vi "Dashboard.Main.vi"() -> ()   [LabVIEW 2014]
uses:
  <vilib>/event_ctls.llb/eventvkey.ctl
  <vilib>/Rock Robotics/WPI/Dashboard/WPI_DashboardLogging Global.vi
  <vilib>/Rock Robotics/Network Tables/SD Read Number.vi
  <vilib>/Rock Robotics/Network Tables/SD Read String.vi
  <vilib>/Rock Robotics/Network Tables/SD Read Boolean.vi
  <vilib>/Rock Robotics/Network Tables/SD Write Number.vi
  <vilib>/Utility/config.llb/Write Key (String).vi
  <vilib>/Utility/config.llb/Write Key (I32).vi
  <vilib>/Utility/config.llb/NI_LVConfig.lvlib
panel:
  in  "TCP":refnum<k5>
  in  "Rec Mode":enum32{"Stop", "Record", "Playback"}(radio)
  in  "Vision":u16(ring) items=["Camera Off", "USB Camera SW", "USB Camera HW", "IP Camera"]
  out "Camera IP":string
  out "Image Message":string="Timeout in Camera Communications"
  in  "Dashboard Tab":T1(tab)=enum."Auto"
  in  "Camera Settings":T2={"Frame Rate"=30, "Compression"=30, "Size"=1} {"Frame Rate" scale=1.0..30.0; "Size" items=["640x480", "320x240", "160x120"]}
  out "MotorChart R":cluster{"Numeric":dbl, "Numeric":dbl}(graph)
  out "MotorChart L":T3(graph)
  out "MotorSliders R":cluster{"MotorSlide1":dbl, "MotorSlide2":dbl} {"MotorSlide2" scale=-1.0..1.0 scale format="%#_2e"; "MotorSlide1" scale=-1.0..1.0 scale format="%#_2e"}
  out "MotorSliders L":T4 {"MotorSlide4 2" scale=0.0..14.0 scale format="%#_2e"; "MotorSlide2" scale=-1.0..1.0 scale format="%#_2e"; "MotorSlide1" scale=-1.0..1.0 scale format="%#_2e"}
  out "Gyro":dbl(knob) scale=0.0..360.0
  out "JS1 Z":dbl(slide) scale=-1.0..1.0 scale format="%#_2e"
  out "JS1 Graph":cluster{"X":dbl, "Y":dbl}[](graph)
  out "JS1 Buttons":T5
  out "JS2 Z":dbl(slide) scale=-1.0..1.0 scale format="%#_2e"
  out "JS2 Graph":cluster{"X":dbl, "Y":dbl}[](graph)
  out "JS2 Buttons":T5
  out "Mode":T6(ring)=enum."Auto Disabled"
  in  "DB Camera Config":bool
  out "fps":dbl format="%#.1g"
  out "Mbps":dbl format="%#.1g"
  out "Mbps 2":bool
  out "Front Detector":bool
  out "Stacker Position":dbl(slide) scale=0.0..20.0
  out "Rear Detector":bool
  out "Current Angle":dbl(knob) scale=0.0..360.0
  out "Commanded Heading":dbl(knob) scale=0.0..360.0
  in  "Auto Selection":T7(radio)
  out "Callback":string
  in  "DB/String 9":string
  in  "DB/String 8":string
  in  "DB/String 7":string
  in  "DB/String 6":string
  in  "DB/String 5":string
  in  "DB/String 4":string
  in  "DB/String 3":string
  in  "DB/String 2":string
  in  "DB/String 1":string
  in  "DB/String 0":string
  in  "DB/Slider 0":dbl(slide) scale=0.0..5.0
  in  "DB/Slider 1":dbl(slide) scale=0.0..5.0
  in  "DB/Slider 2":dbl(slide) scale=0.0..5.0
  in  "DB/Slider 3":dbl(slide) scale=0.0..5.0
  out "DB/LED 3":bool
  out "DB/LED 2":bool
  out "DB/LED 1":bool
  out "DB/LED 0":bool
  in  "DB/Button 3":bool
  in  "DB/Button 2":bool
  in  "DB/Button 1":bool
  in  "DB/Button 0":bool caption="New Name"
  in  "Test Slider":dbl(slide) scale=0.0..100.0 scale format="%#_3g"
  in  "On/Off":bool caption="Solenoid"
  in  "Test Name":u16(ring) items=["Select the test to run...", "Example Test", "-------------------------------", "List of tests is built in robot code.", "Replace with your own automated tests."]
  in  "Test Tree":string(tree)
  in  "Motor":cluster{"Value":dbl, "Enable":bool} {"Value" scale=-1.0..1.0 scale format="%#_3g"}
  out "Progress":T8 {"Test Progress" scale=0.0..100.0}
  in  "Rev/Fwd":cluster{"Forward":bool, "Reverse":bool}
  in  "Test Ring":u16(ring) items=["Monochrome", "Color"]
  in  "Listbox":i32(listbox)
  out "Tree":string(tree)
  out "Camera Image":T9(plugin-control)
  out "Boolean":bool
  # "Left"
  # "Front"
  # "Right"
  # "Battery"
  # "Primary"
  # "Secondary"
  # "Development"
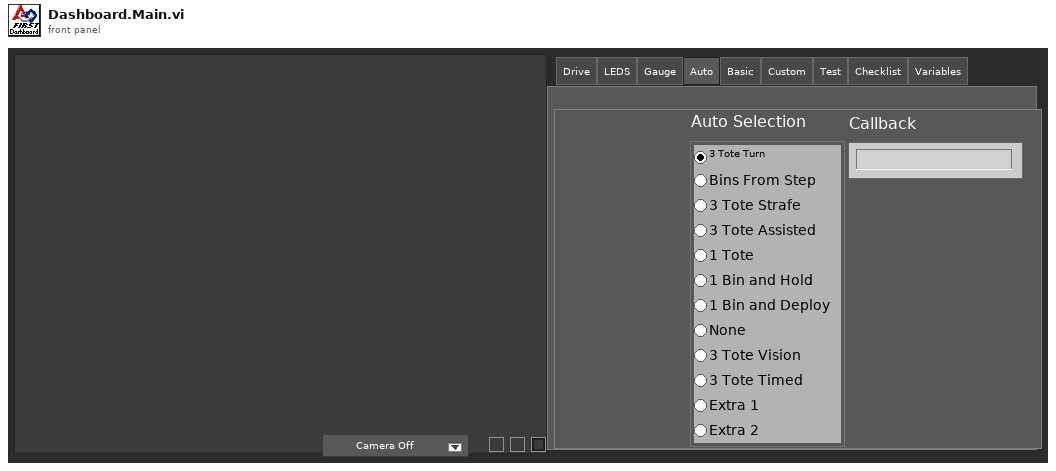
[diagram p1: front panel]
types:
  T1 = enum32{"Drive", "LEDS", "Gauge", "Auto", "Basic", "Custom", "Test", "Checklist", "Variables"}
  T2 = cluster{"Frame Rate":i32, "Compression":i32, "Size":u16}
  T3 = cluster{"Numeric":dbl, "Numeric":dbl, "Battery V":dbl}
  T4 = cluster{"MotorSlide1":dbl, "MotorSlide2":dbl, "MotorSlide4 2":dbl}
  T5 = cluster{bool, bool, bool, bool, bool, bool, bool, bool, bool, bool, bool, bool}
  T6 = enum8{"Tele-Op Disabled", "Tele-Op Enabled", "Auto Disabled", "Auto Enabled", "Test Disabled", "Test Enabled", "Disconnected", "No Code", "E-Stop"}
  T7 = enum32{"3 Tote Turn", "Bins From Step", "3 Tote Strafe", "3 Tote Assisted", "1 Tote", "1 Bin and Hold", "1 Bin and Deploy", "None", "3 Tote Vision", "3 Tote Timed", "Extra 1", "Extra 2"}
  T8 = cluster{"Test Progress":u8, "Test Progress Text":string}
  T9 = typedef "IMAQ Image.ctl" = refnum<image>
  T10 = enum32{"Drive", "Basic", "Custom", "Test", "Checklist", "Variables"}
  T11 = typedef "Image Type" = u32
  T12 = cluster{"Camera Image":refnum<vi>, "Dashboard Tab":refnum<vi>, "Boolean":refnum<vi>, "Vision":refnum<vi>, "Rec Mode":refnum<vi>, "Test Slider":refnum<vi>, "On/Off ":refnum<vi>, "Test Ring":refnum<vi>, "Rev/Fwd":refnum<vi>, "Test Name":refnum<vi>, "Motor":refnum<vi>, "Progress":refnum<vi>, "CheckList":refnum<vi>, "Tree":refnum<vi>, "Test Tree":refnum<vi>}
  T13 = typedef "NI_LVConfig.lvlib/Config Data RefNum.ctl" = refnum<k1>
  T14 = cluster{"Error Strings":string, "Disable Counts":cluster{u16, u16}, "Rail Faults":cluster{u16, u16, u16}, "Robot IP":string, "DB Mode":u8, "Event Info":cluster{"Name":string, "Type":u8, "Number":u16, "Replay":u8}, "Camera Addr":string}
  T15 = cluster{"Storage":cluster{"Disk Free":u64, "RAM Block":u32, "RAM free":u32}, "CPU Utilization":cluster{"CPU % ISR":sgl, "CPU % Time Crit":sgl, "CPU % Timed Str":sgl, "CPU % High":sgl, "CPU % Above":sgl, "CPU % Normal":sgl, "CPU % Low":sgl}, "CAN":cluster{"% Bus Utilization":sgl, "Bus Off Cnt":u32, "TX_FIFO Full Cnt":u32, "Receive Error Cnt":u8, "Transmit Error Cnt":u8}, "HID":cluster{"HID Outputs":u32, "Rumble Low":u16, "Rumble High":u16}[]}
  T16 = cluster{"Status bits":cluster{"Test Mode":bool, "Autonomous":bool, "Enabled":bool, "Code Start":bool, "Brownout":bool, "Reserved 2":bool, "Reserved 3":bool, "E-Stop":bool}, "Code Trace":cluster{"Disabled":bool, "TeleOp":bool, "Auto":bool, "Test":bool}, "Controller Type":enum16{"unknown", "cRIO", "roboRio"}, "Code?":enum16{"unknown", "noCode", "code"}, "Battery V":dbl}
  T17 = cluster{"Control Bits":cluster{"TestMode":bool, "Autonomous":bool, "Enabled":bool, "FMS Present":bool, bool, bool, bool, "E-Stop":bool}, "Team Station ":u8, "Countdown":sgl, "Joystick Values":cluster{"Axes":dbl[], "Buttons":bool[], "POVs":i16[]}[]}
  T18 = cluster{"Axes":dbl[], "Buttons":bool[], "POVs":i16[]}[]
  T19 = cluster{"Axes":dbl[], "Buttons":bool[], "POVs":i16[]}
  T20 = cluster{"Buttons[0]":bool, "Buttons[1]":bool, "Buttons[2]":bool, "Buttons[3]":bool, "Buttons[4]":bool, "Buttons[5]":bool, "Buttons[6]":bool, "Buttons[7]":bool, "Buttons[8]":bool, "Buttons[9]":bool, "Buttons[10]":bool, "Buttons[11]":bool}
  T21 = cluster{"Operation":enum16{"Update", "Clear"}, "Color Box":u32}[]
  T22 = typedef "eventvkey.ctl" = enum16{"ASCII", "Enter", "Return", "Shift", "Ctrl", "Alt", "Cmd", "Opt", "Caps", "NumLock", "Clear", "Break", "Up", "Down", "Left", "Right", "Insert", "Delete", "Home", "End", "PageUp", "PageDown", "Escape", "Help", "Pause", "ScrollLock", "F1", "F2", "F3", "F4", "F5", "F6", "F7", "F8", "F9", "F10", "F11", "F12", "F13", "F14", "F15", "F16", "F17", "F18", "F19", "F20", "F21", "F22", "F23", "F24", "Play", "VolumeUp", "VolumeDown", "Mute", "Two Byte Char"}
  T23 = cluster{"Image Size":bool, "Image Type":bool, "Pixel Value":bool, "ROI Information":bool, "Zoom Factor":bool}
  T24 = enum8{"Enabled", "Disabled", "Disabled and Grayed Out"}
  T25 = cluster{"Operation":enum16{"Update", "Clear"}, "Color Box":u32}
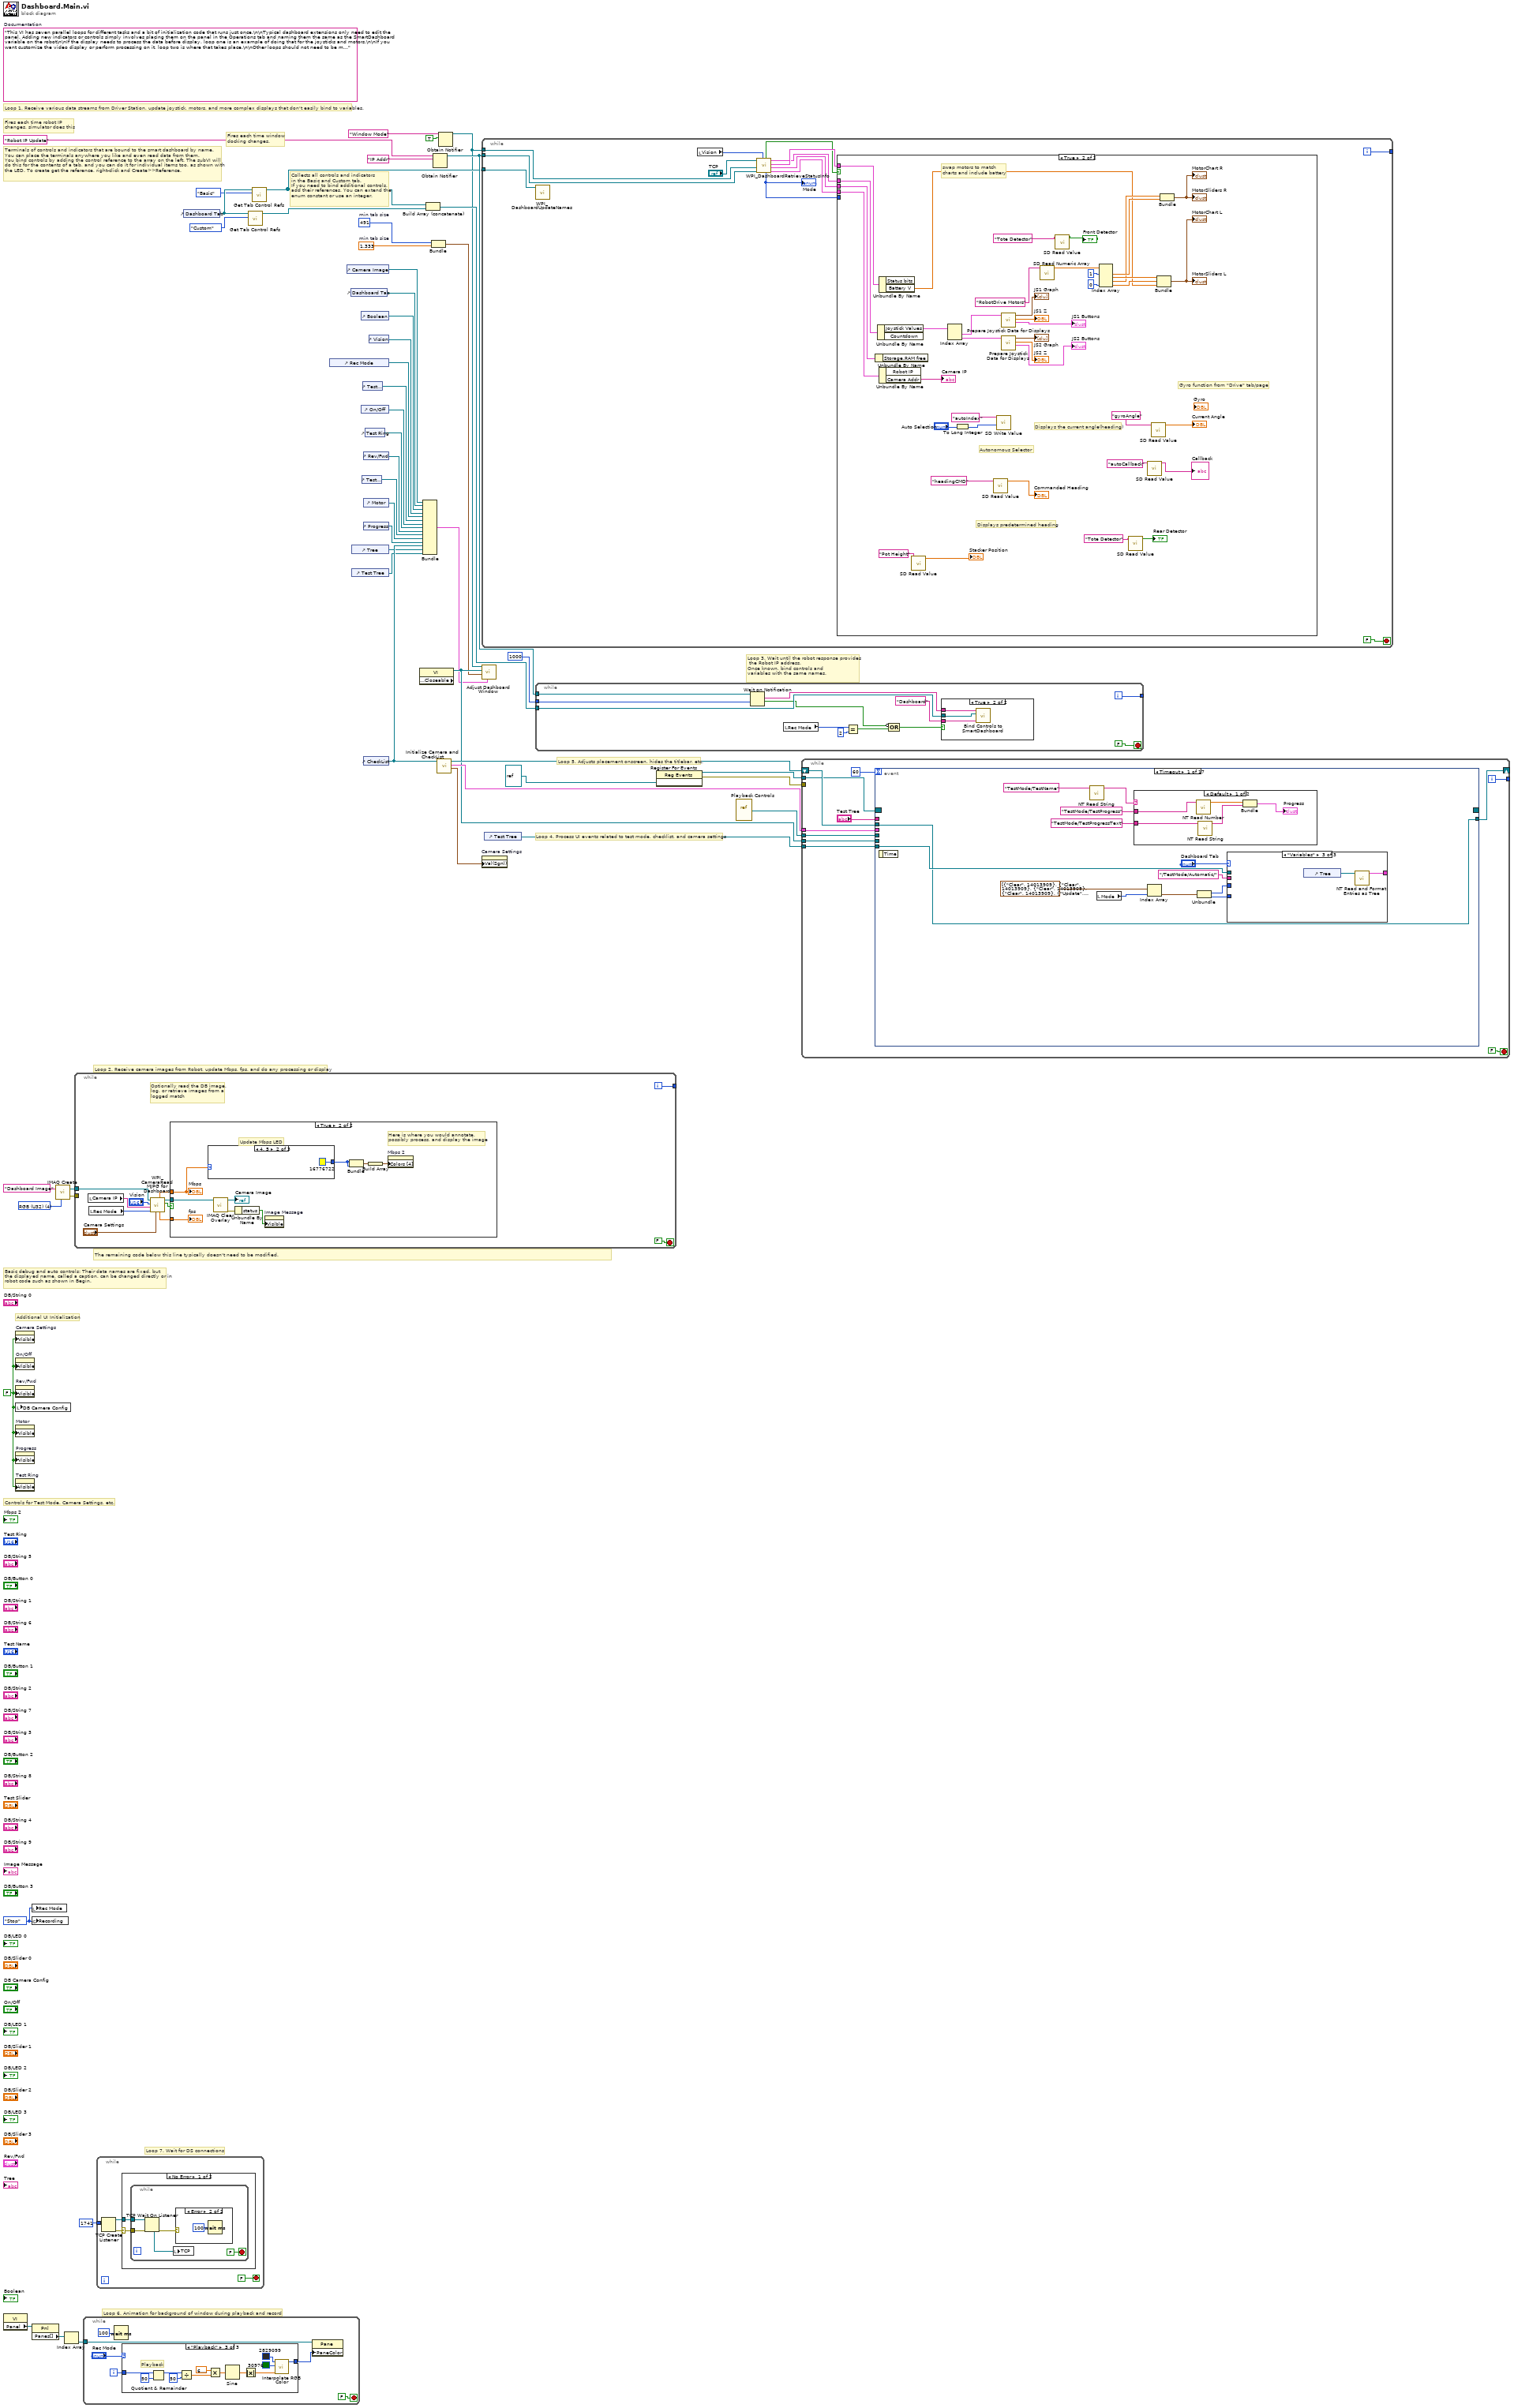
[diagram p0: block diagram]
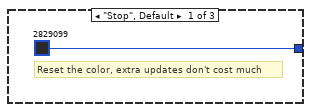
[diagram p5: hidden frame]
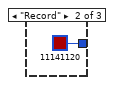
[diagram p6: hidden frame]
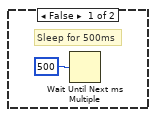
[diagram p8: hidden frame]
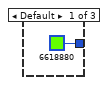
[diagram p9: hidden frame]
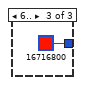
[diagram p10: hidden frame]
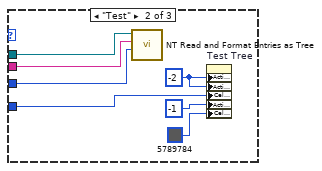
[diagram p12: hidden frame]
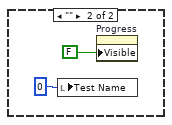
[diagram p13: hidden frame]
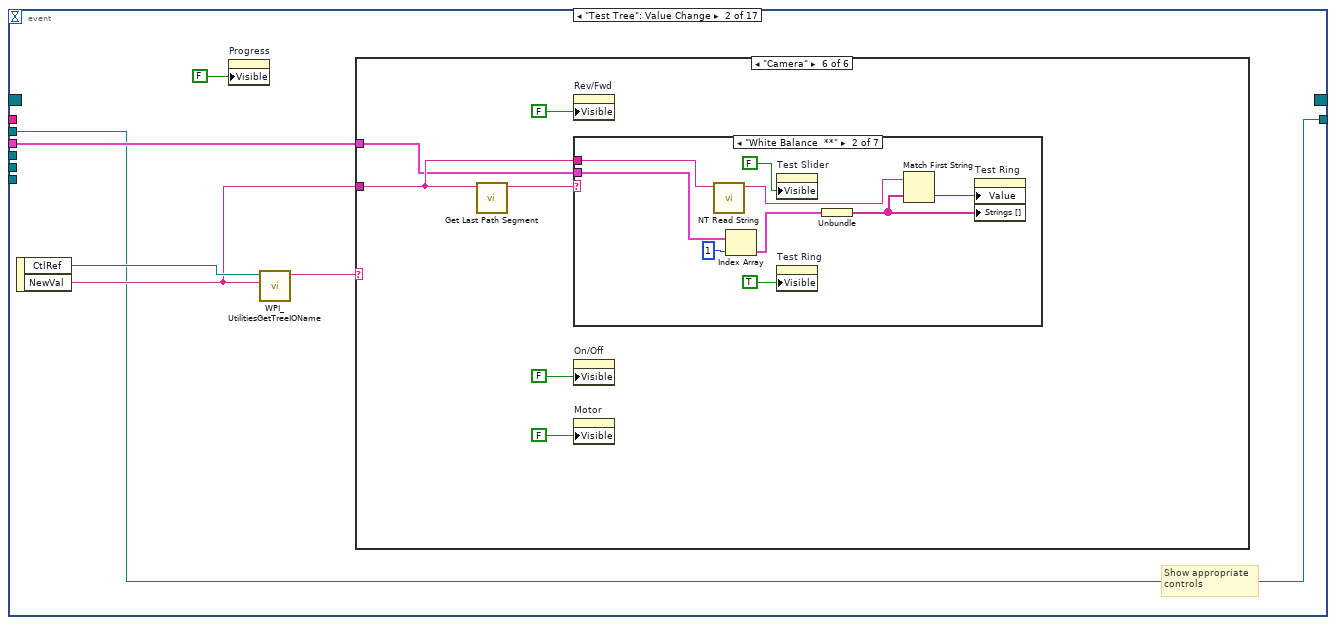
[diagram p14: hidden frame]
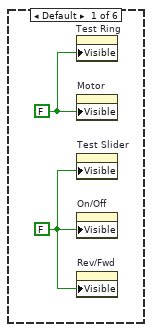
[diagram p15: hidden frame]
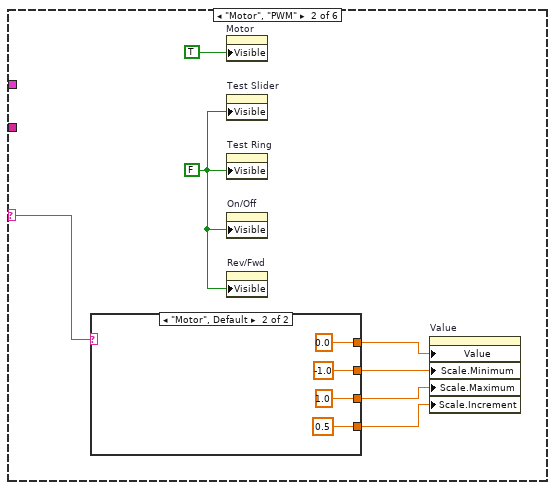
[diagram p16: hidden frame]
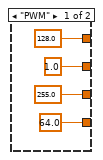
[diagram p17: hidden frame]
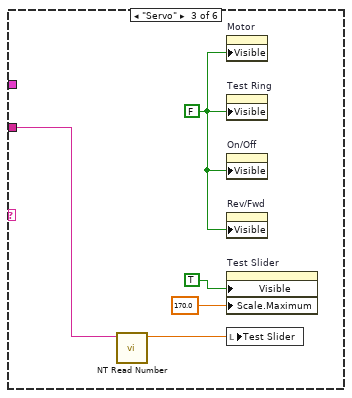
[diagram p18: hidden frame]
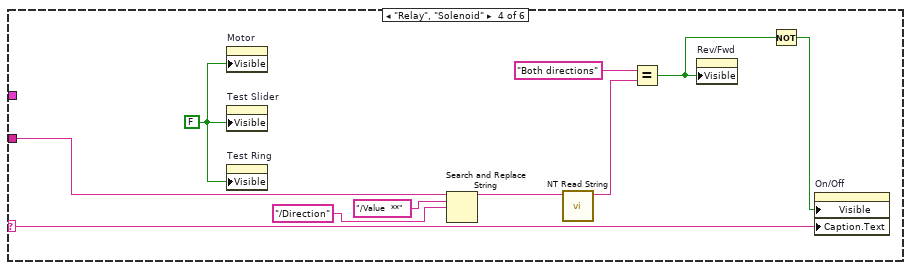
[diagram p19: hidden frame]
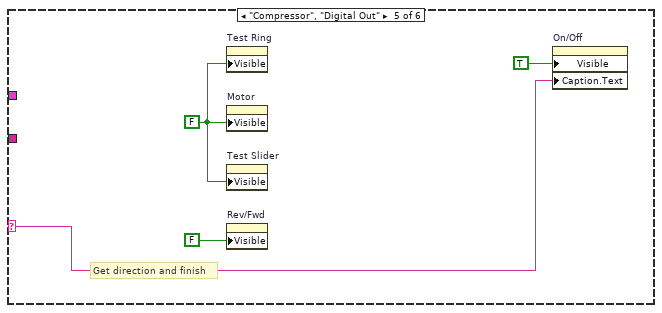
[diagram p20: hidden frame]
diagram:
  w23 = 491  # min tab size
  w22 = 1.333  # min tab size
  w31 = enum32{"Stop", "Record", "Playback"}."Stop" ("Rec Mode")
  w5 = FALSE ("Visible")
  (unwired) "This VI has seven parallel loops for different tasks and a bit of initialization code that runs just once.\n\nTypical dashboard extensions only need to edit the panel. Adding new indicators or controls simply involves placing them on the panel in the Operations tab and naming them the same as the SmartDashboard variable on the robot\n\nIf the display needs to process the data before display, loop one is an example of doing that for the joysticks and motors.\n\nIf you want customize the video display or perform processing on it, loop two is where that takes place.\n\nOther loops should not need to be modified. They are pretty standard, and document the task they perform."  # Documentation
  w51 = T11 4 items=["Grayscale (U8)", "Grayscale (I16)", "Grayscale (SGL)", "Complex (CSG)", "RGB (U32)", "HSL (U32)", "RGB (U64)"] ("Image Type")
  # "Loop 7. Wait for DS connections"
  # "Basic debug and auto controls: Their data names are fixed, but\nthe displayed name, called a caption, can be changed directly or in\nrobot code such as shown in Begin."
  # "Controls for Test Mode, Camera Settings, etc."
  # "Additional UI Initialization"
  # "Loop 6. Animation for background of window during playback and record"
  # "Fires each time robot IP\nchanges, simulator does this"
  # "Fires each time window\ndocking changes."
  # "Collects all controls and indicators\nin the Basic and Custom tab.\nIf you need to bind additional controls,\nadd their references. You can extend the\nenum constant or use an integer."
  # "The remaining code below this line typically doesn't need to be modified."
  # "Loop 4. Process UI events related to test mode, checklist, and camera settings"
  # "Terminals of controls and indicators that are bound to the smart dashboard by name.\nYou can place the terminals anywhere you like and even read data from them.\nYou bind controls by adding the control reference to the array on the left. The subVI will\ndo this for the contents of a tab, and you can do it for individual items too, as shown with\nthe LED. To create get the reference, right-click and Create>>Reference."
  # "Loop 3. Wait until the robot response provides\n the Robot IP address.\nOnce known, bind controls and\nvariables with the same names."
  # "Loop 5. Adjusts placement onscreen, hides the titlebar, etc."
  # "Loop 1. Receive various data streams from Driver Station, update joystick, motors, and more complex displays that don't easily bind to variables."
  # "Loop 2. Receive camera images from Robot, update Mbps, fps, and do any processing or display"
  n1 = property class="VI"() -> ("Panel"=w38:refnum<vi>)  [unwired: 2 in, 2 out]
  n2 = property on="Camera Settings" class="Clust (strict)"("Visible"=w5) -> ()  [unwired: 2 in, 2 out]
  n3 = property on="On/Off" class="Bool (strict)"("Visible"=w5) -> ()  [unwired: 2 in, 2 out]
  n4 = property on="Rev/Fwd" class="Clust (strict)"("Visible"=w5) -> ()  [unwired: 2 in, 2 out]
  n5 = local write "DB Camera Config"(w5) -> ()
  n6 = property on="Motor" class="Clust (strict)"("Visible"=w5) -> ()  [unwired: 2 in, 2 out]
  n7 = property on="Progress" class="Clust (strict)"("Visible"=w5) -> ()  [unwired: 2 in, 2 out]
  n8 = property on="Test Ring" class="Ring (strict)"("Visible"=w5) -> ()  [unwired: 2 in, 2 out]
  n9 = local write "Rec Mode"(w31) -> ()
  n10 = global write "WPI_DashboardLogging Global.vi" "Recording"(w31) -> ()
  n11 = property class="Pnl"(reference=w38) -> ("Panes[]"=w39:refnum<vi>[])  [unwired: 1 in, 2 out]
  n12 = call "IMAQ Create"("Image Name"="Dashboard Image", "Image Type"=w51) -> ("New Image"=w49:T9, "error out"=w48:errorcluster)  [unwired: 2 in, 1 out]
  n13 = Index Array(array=w39) -> (element=w37:refnum<vi>)  [unwired: 1 in]
  n14 = while {
    tunnel: w49 -> [w60]
    tunnel: w48 -> [_]
    tunnel: [w61] -> _
    i -> [w61]
    stop <- FALSE stop-if-true
    # "Optionally read the DB image,\nlog, or retrieve images from a\nlogged match"
    n15 = local read "Camera IP"() -> (w52:string)
    n16 = local read "Rec Mode"() -> (w54:enum32{"Stop", "Record", "Playback"})
    n17 = call <vilib>:"WPI_CameraRead MJPG for Dashboard.vi"("Camera Settings"="Camera Settings", "Rec Mode"=w54, "Camera IP"=w52, "Camera Mode"="Vision", "Refnum in"=w60) -> ("Active"=w58:bool, "Refnum out"=w59:T9, "FPS"=w57:dbl, "Bandwidth (Mbps)"=w56:dbl)  [unwired: 3 in]
    n18 = case shown="True" w58 {
      tunnel: w59 -> [_ w67]
      tunnel: w56 -> [_ w66]
      tunnel: w57 -> [_ w64]
      frame False {
        # "Sleep for 500ms"
        n19 = Wait Until Next ms Multiple(millisecond multiple=u32 500) -> ()  [unwired: 1 out]
      }
      frame True {
        # "Here is where you would annotate,\npossibly process, and display the image"
        # "Update Mbps LED"
        n20 = case shown="4, 5" w66 {
          tunnel: [u32 6618880 ("Color Box") u32 16776722 ("Color Box") u32 16716800 ("Color Box")] -> w68
          frame Default {
          }
          frame 4, 5 {
          }
          frame 6.. {
          }
        }
        n21 = call "IMAQ Clear Overlay"("Image"=w67) -> ("error out"=w71:errorcluster, "Image Out"=→"Camera Image":T9)  [unwired: 2 in, 7 out]
        n22 = Unbundle By Name(w71) -> ("status"=w72:bool)
        n23 = property on="Image Message" class="Str"("Visible"=w72) -> ()  [unwired: 2 in, 2 out]
        n24 = Bundle("Color Box"=w68, "Color Box"=w68) -> (w70:cluster{"Color Box":u32, "Color Box":u32})  [unwired: 1 out]
        n25 = Build Array(w70) -> (w69:cluster{"Color Box":u32, "Color Box":u32}[])
        n26 = property on="Mbps 2" class="Bool (strict)"("Colors [4]"=w69) -> ()  [unwired: 2 in, 2 out]
        "Mbps" <- w66
        "fps" <- w64
      }
    }
  }
  n27 = while {
    tunnel: w37 -> [w77]
    i -> [w80]
    stop <- FALSE stop-if-true
    n28 = Wait (ms)(milliseconds to wait=u32 100) -> ()  [unwired: 1 out]
    n29 = case shown="\"Playback\"" "Rec Mode" {
      tunnel: w80 -> [_ _ w95]
      tunnel: [u32 2829099 ("Base Color") u32 11141120 ("Target Color") w84] -> w76
      frame "Stop", Default {
        # "Reset the color, extra updates don't cost much"
      }
      frame "Record" {
      }
      frame "Playback" {
        # "Playback"
        n30 = Quotient & Remainder(x=w95, y=u32 50 ("milliseconds to wait")) -> (x-y*floor(x/y)=w91:u32)  [unwired: 1 out]
        n31 = Divide(x=w91, y=u32 50 ("milliseconds to wait")) -> (x/y=w88:dbl)
        n32 = Multiply(x=6.283185307179586, y=w88) -> (x*y=w93:dbl)
        n33 = Sine(x=w93) -> (sin(x)=w92:dbl)
        n34 = Absolute Value(x=w92) -> (abs(x)=w85:dbl)
        n35 = call "Interpolate RGB Color.vi"("Proportion"=w85, "Target Color"=u32 30976, "Base Color"=u32 2829099) -> ("Result Color"=w84:u32)  [unwired: 8 in]
      }
    }
    n36 = property class="Pane"(reference=w77, "PaneColor"=w76) -> ()  [unwired: 1 in, 2 out]
  }
  n37 = while {
    tunnel: u16 1741 ("timeout ms (25000)") -> [w99]
    stop <- FALSE stop-if-true
    n38 = TCP Create Listener(10:w99) -> (0:w96:errorcluster, 3:w98:refnum<k5>)  [unwired: 4 in, 1 out]
    n39 = case shown="No Error" w96 {
      selector: w96 -> [w100 _]
      tunnel: w98 -> [w101 _]
      frame No Error {
        n40 = while {
          tunnel: w101 -> [w105]
          tunnel: w100 -> [w103]
          stop <- FALSE stop-if-true
          n41 = TCP Wait On Listener(8:w103, 11:w105) -> (0:w102:errorcluster, 4:w104:refnum<k5>)  [unwired: 2 in, 3 out]
          n42 = local write "TCP"(w104) -> ()
          n43 = case shown="Error" w102 {
            frame No Error {
            }
            frame Error {
              n44 = Wait (ms)(milliseconds to wait=u32 100) -> ()  [unwired: 1 out]
            }
          }
        }
      }
      frame Error {
      }
    }
  }
  n45 = control-ref of="Dashboard Tab"() -> (w29:refnum<vi>)
  n46 = call <vilib>:"Get Tab Control Refs.vi"("Page Index"=T10."Custom" ("Dashboard Tab"), "TabControl in"=w29) -> ("ControlsOnPage"=w28:refnum<vi>[])  [unwired: 9 in]
  n47 = call <vilib>:"Get Tab Control Refs.vi"("Page Index"=T10."Basic" ("Dashboard Tab"), "TabControl in"=w29) -> ("ControlsOnPage"=w3:refnum<vi>[])  [unwired: 9 in]
  n48 = control-ref of="Rec Mode"() -> (w11:refnum<vi>)
  n49 = control-ref of="Camera Image"() -> (w26:refnum<vi>)
  n50 = control-ref of="Dashboard Tab"() -> (w25:refnum<vi>)
  n51 = control-ref of="Tree"() -> (w15:refnum<vi>)
  n52 = control-ref of="Test Tree"() -> (w14:refnum<vi>)
  n53 = control-ref of="Boolean"() -> (w20:refnum<vi>)
  n54 = control-ref of="On/Off"() -> (w9:refnum<vi>)
  n55 = control-ref of="Test Name"() -> (w13:refnum<vi>)
  n56 = control-ref of="Test Slider"() -> (w10:refnum<vi>)
  n57 = control-ref of="Rev/Fwd"() -> (w7:refnum<vi>)
  n58 = control-ref of="Motor"() -> (w12:refnum<vi>)
  n59 = control-ref of="Progress"() -> (w6:refnum<vi>)
  n60 = control-ref of="CheckList"() -> (w16:refnum<vi>)
  n61 = control-ref of="Test Ring"() -> (w8:refnum<vi>)
  n62 = control-ref of="Vision"() -> (w24:refnum<vi>)
  n63 = property class="VI" props=["Front Panel.Closeable"]() -> (reference out=w30:refnum<vi>)  [unwired: 2 in, 2 out]
  n64 = Bundle("Camera Image"=w26, "Dashboard Tab"=w25, "Boolean"=w20, "Vision"=w24, "Rec Mode"=w11, "Test Slider"=w10, "On/Off"=w9, "Test Ring"=w8, "Rev/Fwd"=w7, "Test Name"=w13, "Motor"=w12, "Progress"=w6, "CheckList"=w16, "Tree"=w15, "Test Tree"=w14) -> (w17:T12)  [unwired: 1 in]
  n65 = Build Array (concatenate)(w3, w28) -> (w27:refnum<vi>[])
  n66 = Bundle("min tab size"=w23, "min tab size"=w22) -> (w21:cluster{"min tab size":i32, "min tab size":dbl})  [unwired: 1 in]
  n67 = Obtain Notifier(name (unnamed)="Robot IP Update", notification data type="IP Addr" ("name (unnamed)")) -> (notifier out=w4:refnum<notifier>)  [unwired: 2 in, 2 out]
  n68 = call "Initialize Camera and CheckList.vi"("ListBox in"=w16) -> ("Cluster"=w42:cluster{"value":i32, "value":i32, "index":i32}, "Array"=w43:cluster{string[]}[], "File Refnum"=w41:T13)  [unwired: 8 in]
  n69 = Obtain Notifier(name (unnamed)="Window Mode", notification data type=TRUE) -> (notifier out=w2:refnum<notifier>)  [unwired: 2 in, 2 out]
  n70 = while {
    tunnel: [w119] -> _
    tunnel: w4 -> [w113]
    tunnel: w3 -> [w112]
    tunnel: w2 -> [w108]
    i -> [w119]
    stop <- FALSE stop-if-true
    n71 = call <vilib>:"WPI_DashboardUpdateNames.vi"("Controls on Tab"=w112) -> ()  [unwired: 11 in]
    n72 = local read "Vision"() -> (w110:u16)
    n73 = call <vilib>:"WPI_DashboardRetrieveStatusInfo.vi"("Vision"=w110, "Binding Refnum"=w113, "Window Mode Notifier"=w108, "TCP Cnx"="TCP") -> ("Power and Errors"=w114:T14, "Robot Metrics"=w117:T15, "Status Info"=w118:T16, "Control Info"=w115:T17, "Robot Mode"=w111:T6, "Process?"=w116:bool)  [unwired: 2 in]
    "Mode" <- w111
    n74 = case shown="True" w116 {
      tunnel: w118 -> [_ w160]
      tunnel: w117 -> [_ w159]
      tunnel: w115 -> [_ w158]
      tunnel: w114 -> [_ w157]
      tunnel: w111 -> [_ _]
      frame False {
      }
      frame True {
        # "Gyro function from \"Drive\" tab/page"
        # "Displays the current angle(heading)"
        # "Displays predetermined heading"
        # "Autonomous Selector"
        # "swap motors to match\ncharts and include battery"
        n75 = Unbundle By Name(w159) -> ()  [unwired: 1 out]
        n76 = Unbundle By Name(w158) -> ("Joystick Values"=w145:T18)  [unwired: 1 out]
        n77 = Unbundle By Name(w157) -> ("Camera Addr"=→"Camera IP":string)  [unwired: 1 out]
        n78 = Unbundle By Name(w160) -> ("Battery V"=w146:dbl)  [unwired: 1 out]
        n79 = call-poly <vilib>:"SD Read Value.vi"("Name"="Pot Height") -> ("Numeric"=→"Stacker Position":dbl)  [unwired: 8 in, 2 out]
        n80 = Index Array(array=w145) -> (element #1=w144:T19, element #2=w139:T19)  [unwired: 2 in]
        n81 = To Long Integer(number="Auto Selection") -> (32bit integer=w121:i32)
        n82 = call-poly <vilib>:"SD Read Value.vi"("Name"="headingCMD") -> ("Numeric"=→"Commanded Heading":dbl)  [unwired: 8 in, 2 out]
        n83 = call-poly <vilib>:"SD Write Value.vi"("Numeric"=w121, "Name"="autoIndex") -> ()  [unwired: 8 in, 2 out]
        n84 = call "Prepare Joystick Data for Displays.vi"("Joystick Values"=w144) -> ("Buttons"=→"JS1 Buttons":T20, "Z Axis"=→"JS1 Z":dbl, "Cartesian Data"=→"JS1 Graph":cluster{"X axis":dbl, "X axis":dbl}[])  [unwired: 8 in]
        n85 = call "Prepare Joystick Data for Displays.vi"("Joystick Values"=w139) -> ("Buttons"=→"JS2 Buttons":T20, "Z Axis"=→"JS2 Z":dbl, "Cartesian Data"=→"JS2 Graph":cluster{"X axis":dbl, "X axis":dbl}[])  [unwired: 8 in]
        n86 = call <vilib>:"SD Read Numeric Array.vi"("Name"="RobotDrive Motors") -> ("Numeric Array"=w148:dbl[])  [unwired: 8 in, 2 out]
        n87 = call-poly <vilib>:"SD Read Value.vi"("Name"="Tote Detector") -> ("Boolean"=→"Front Detector":bool)  [unwired: 8 in, 2 out]
        n88 = Index Array(array=w148, index #1=1, index #4=0) -> (element #1=w152:dbl, element #2=w153:dbl, element #3=w151:dbl, element #4=w156:dbl)  [unwired: 2 in]
        n89 = call-poly <vilib>:"SD Read Value.vi"("Name"="Tote Detector") -> ("Boolean"=→"Rear Detector":bool)  [unwired: 8 in, 2 out]
        n90 = call-poly <vilib>:"SD Read Value.vi"("Name"="autoCallback") -> ("String"=→"Callback":string)  [unwired: 8 in, 2 out]
        n91 = call-poly <vilib>:"SD Read Value.vi"("Name"="gyroAngle") -> ("Numeric"=→"Current Angle":dbl)  [unwired: 8 in, 2 out]
        n92 = Bundle("Numeric"=w153, "Numeric"=w156, "Battery V"=w146) -> (→"MotorChart L" →"MotorSliders L":T3)  [unwired: 1 in]
        n93 = Bundle("Numeric"=w151, "Numeric"=w152) -> (→"MotorChart R" →"MotorSliders R":cluster{"Numeric":dbl, "Numeric":dbl})  [unwired: 1 in]
      }
    }
  }
  n94 = call "Adjust Dashboard Window.vi"("Sizing Refnums"=w17, "Size Constraints"=w21, "VI"=w30, "Notifier in"=w2) -> ()  [unwired: 8 in]
  n95 = property on="Camera Settings" class="Clust (strict)"("Val(Sgnl)"=w42) -> ()  [unwired: 2 in, 2 out]
  n96 = control-ref of="Test Tree"() -> (w40:refnum<vi>)
  n97 = while {
    tunnel: w27 -> [w172]
    tunnel: w4 -> [w170]
    tunnel: [w168] -> _
    tunnel: u32 1000 ("milliseconds to wait") -> [w167]
    i -> [w168]
    stop <- FALSE stop-if-true
    n98 = Wait on Notification(notifier=w170, timeout in ms (-1)=w167) -> (notification=w169:string, timed out?=w165:bool)  [unwired: 2 in, 2 out]
    n99 = local read "Rec Mode"() -> (w163:enum32{"Stop", "Record", "Playback"})
    n100 = Equal?(x=w163, y=u16 2 ("Rec Mode")) -> (x = y?=w164:bool)
    n101 = Compound Arithmetic op=OR(invert w165, w164) -> (w166:bool)
    n102 = case shown="True" w166 {
      tunnel: w172 -> [_ w175]
      tunnel: w169 -> [_ w174]
      tunnel: "Dashboard" -> [_ w173]
      frame False {
      }
      frame True {
        n103 = call <vilib>:"Bind Controls to SmartDashboard.vi"("Client Name"=w173, "Bound Control Refs"=w175, "Server IP Address"=w174) -> ()  [unwired: 9 in]
      }
    }
  }
  n104 = register-events(refnum<vi> refnum) -> (reference out=w35:refnum<event-registration>, error out=w34:errorcluster)  [unwired: 2 in]
  n105 = vi-ref "Playback Controls.vi"() -> (w36:refnum<vi>)
  n106 = while {
    tunnel: w43 -> [w183]
    shift-right: [w182] -> _
    shift-left: w41 -> [w181]
    tunnel: [w180] -> _
    tunnel: w40 -> [w179]
    tunnel: w36 -> [w178]
    tunnel: w35 -> [w177]
    tunnel: w34 -> [_]
    tunnel: w30 -> [w176]
    i -> [w180]
    stop <- FALSE stop-if-true
    n107 = event shown="[0] Timeout" {
      selector: w177 -> [_ _ _ _ _ _ _ _ _ _ _ _ _ _ _ _ _]
      dyn-events: [_ _ _ _ _ _ _ _ _ _ _ _ _ w421 _ _ _] -> _
      timeout: u32 60 ("milliseconds to wait") -> [_ _ _ _ _ _ _ _ _ _ _ _ _ _ _ _ _]
      tunnel: w179 -> [w195 _ _ _ _ _ _ _ _ _ _ _ _ _ _ _ _]
      tunnel: "Test Tree" -> [_ _ _ _ _ _ _ _ w390 w398 w400 w404 w412 _ _ _ _]
      tunnel: w183 -> [_ w217 _ _ _ _ w354 w384 _ _ _ _ _ _ _ _ _]
      tunnel: [w191 w216 w315 w320 w328 w340 w353 w377 w389 w396 w399 w403 w411 w423 w437 w438 w448] -> w182
      tunnel: w181 -> [w191 w216 w315 w320 w328 w340 w352 w377 w389 w396 w399 w403 w411 w423 w437 w438 w448]
      tunnel: w178 -> [_ _ _ _ _ _ _ _ _ _ _ _ _ w424 _ w441 _]
      tunnel: w176 -> [_ _ _ _ _ _ _ _ _ _ _ _ _ w419 _ _ _]
      event Timeout {
        n108 = event-data() -> ()  [unwired: 1 in, 1 out]
        n109 = call <vilib>:"NT Read String.vi"("Name"="TestMode/TestName") -> ("String"=w198:string)  [unwired: 9 in, 1 out]
        n110 = local read "Mode"() -> (w194:T6)
        n111 = case shown="Default" w198 {
          tunnel: "TestMode/TestProgress" ("Name") -> [w210 _]
          tunnel: "TestMode/TestProgressText" ("Name") -> [w209 _]
          frame Default {
            n112 = call <vilib>:"NT Read Number.vi"("Name"=w210) -> ("Numeric"=w211:dbl)  [unwired: 9 in, 1 out]
            n113 = call <vilib>:"NT Read String.vi"("Name"=w209) -> ("String"=w212:string)  [unwired: 9 in, 1 out]
            n114 = Bundle("Numeric"=w211, "String"=w212) -> (→"Progress":cluster{"Numeric":dbl, "String":string})  [unwired: 1 in]
          }
          frame "" {
            n115 = local write "Test Name"(u16 0) -> ()
            n116 = property on="Progress" class="Clust (strict)"("Visible"=FALSE) -> ()  [unwired: 2 in, 2 out]
          }
        }
        n117 = Index Array(array=T21 [{"Operation"=enum."Clear", "Color Box"=14013909}, {"Operation"=enum."Clear", "Color Box"=14013909}, {"Operation"=enum."Clear", "Color Box"=14013909}, {"Operation"=enum."Clear", "Color Box"=14013909}, {"Operation"=enum."Update", "Color Box"=14013909}, {"Operation"=enum."Update", "Color Box"=16777215}, {"Operation"=enum."Clear", "Color Box"=14013909}, {"Operation"=enum."Clear", "Color Box"=14013909}, {"Operation"=enum."Clear", "Color Box"=14013909}], index=w194) -> (element=w189:T25)
        n118 = Unbundle(w189) -> ("Operation"=w188:enum16{"Update", "Clear"}, "Color Box"=w187:u32)
        n119 = case shown="\"Variables\"" "Dashboard Tab" {
          tunnel: w195 -> [_ w206 _]
          tunnel: "/TestMode/Automatic/" ("Name Pattern") -> [_ w205 _]
          tunnel: w188 -> [_ w204 _]
          tunnel: [_ _ w208] -> _
          tunnel: w187 -> [_ w200 _]
          frame "Custom", Default {
          }
          frame "Test" {
            w203 = -2 ("Active Item:Row Number")
            n120 = call <vilib>:"NT Read and Format Entries as Tree.vi"("Operation"=w204, "Name Pattern"=w205, "Tree Refnum"=w206) -> ()  [unwired: 7 in, 2 out]
            n121 = property on="Test Tree" class="Tree (strict)"("Active Item Row Number"=w203, "ActiveColNum"=w203, "CellBG"=w200, "Active Item Row Number"=-1 ("Active Item:Row Number"), "CellBG"=u32 5789784 ("Color Box")) -> ()  [unwired: 2 in, 2 out]
          }
          frame "Variables" {
            n122 = control-ref of="Tree"() -> (w207:refnum<vi>)
            n123 = call <vilib>:"NT Read and Format Entries as Tree.vi"("Tree Refnum"=w207) -> ("Formatted Strings"=w208:cluster{"Name":string, "Value":string}[])  [unwired: 9 in, 1 out]
          }
        }
      }
      event "Test Tree": Value Change {
        # "Show appropriate\ncontrols"
        n124 = event-data() -> ("CtlRef"=w220:refnum<vi>, "NewVal"=w218:string)  [unwired: 1 in]
        n125 = property on="Progress" class="Clust (strict)"("Visible"=FALSE) -> ()  [unwired: 2 in, 2 out]
        n126 = call <vilib>:"WPI_UtilitiesGetTreeIOName.vi"("NewVal"=w218, "TreeControl in"=w220) -> ("I/O Name"=w221:string)  [unwired: 9 in]
        n127 = case shown="\"Camera\"" w221 {
          selector: w221 -> [_ w228 _ w246 w255 _]
          tunnel: w218 -> [_ _ w243 w245 _ w262]
          tunnel: w217 -> [_ _ _ _ _ w261]
          frame Default {
            w223 = FALSE ("Visible")
            w222 = FALSE ("Visible")
            n128 = property on="Test Ring" class="Ring (strict)"("Visible"=w222) -> ()  [unwired: 2 in, 2 out]
            n129 = property on="Motor" class="Clust (strict)"("Visible"=w222) -> ()  [unwired: 2 in, 2 out]
            n130 = property on="Test Slider" class="Slide (strict)"("Visible"=w223) -> ()  [unwired: 2 in, 2 out]
            n131 = property on="On/Off" class="Bool (strict)"("Visible"=w223) -> ()  [unwired: 2 in, 2 out]
            n132 = property on="Rev/Fwd" class="Clust (strict)"("Visible"=w223) -> ()  [unwired: 2 in, 2 out]
          }
          frame "Motor", "PWM" {
            w229 = FALSE ("Visible")
            n133 = case shown="\"Motor\", Default" w228 {
              tunnel: [1.0 ("Value") -1.0 ("Value")] -> w227
              tunnel: [255.0 ("Value") 1.0 ("Value")] -> w226
              tunnel: [128.0 ("Value") 0.0 ("Value")] -> w225
              tunnel: [64.0 ("Value") 0.5 ("Value")] -> w224
              frame "PWM" {
              }
              frame "Motor", Default {
              }
            }
            n134 = property on="Motor" class="Clust (strict)"("Visible"=TRUE) -> ()  [unwired: 2 in, 2 out]
            n135 = property on="Test Slider" class="Slide (strict)"("Visible"=w229) -> ()  [unwired: 2 in, 2 out]
            n136 = property on="Test Ring" class="Ring (strict)"("Visible"=w229) -> ()  [unwired: 2 in, 2 out]
            n137 = property on="On/Off" class="Bool (strict)"("Visible"=w229) -> ()  [unwired: 2 in, 2 out]
            n138 = property on="Rev/Fwd" class="Clust (strict)"("Visible"=w229) -> ()  [unwired: 2 in, 2 out]
            n139 = property on="Value" class="Slide (strict)"("Value"=w225, "Scale.Minimum"=w227, "Scale.Maximum"=w226, "Scale.Increment"=w224) -> ()  [unwired: 2 in, 2 out]
          }
          frame "Servo" {
            w241 = FALSE ("Visible")
            n140 = call <vilib>:"NT Read Number.vi"("Name"=w243) -> ("Numeric"=w242:dbl)  [unwired: 9 in, 1 out]
            n141 = property on="Motor" class="Clust (strict)"("Visible"=w241) -> ()  [unwired: 2 in, 2 out]
            n142 = property on="Test Ring" class="Ring (strict)"("Visible"=w241) -> ()  [unwired: 2 in, 2 out]
            n143 = property on="On/Off" class="Bool (strict)"("Visible"=w241) -> ()  [unwired: 2 in, 2 out]
            n144 = property on="Rev/Fwd" class="Clust (strict)"("Visible"=w241) -> ()  [unwired: 2 in, 2 out]
            n145 = property on="Test Slider" class="Slide (strict)"("Visible"=TRUE, "Scale.Maximum"=170.0 ("Scale.Range:Maximum")) -> ()  [unwired: 2 in, 2 out]
            n146 = local write "Test Slider"(w242) -> ()
          }
          frame "Relay", "Solenoid" {
            w244 = FALSE ("Visible")
            n147 = property on="Motor" class="Clust (strict)"("Visible"=w244) -> ()  [unwired: 2 in, 2 out]
            n148 = property on="Test Slider" class="Slide (strict)"("Visible"=w244) -> ()  [unwired: 2 in, 2 out]
            n149 = property on="Test Ring" class="Ring (strict)"("Visible"=w244) -> ()  [unwired: 2 in, 2 out]
            n150 = Search and Replace String(input string=w245, search string="/Value  **", replace string="/Direction") -> (result string=w251:string)  [unwired: 5 in, 3 out]
            n151 = call <vilib>:"NT Read String.vi"("Name"=w251) -> ("String"=w249:string)  [unwired: 9 in, 1 out]
            n152 = Equal?(x="Both directions", y=w249) -> (x = y?=w247:bool)
            n153 = property on="Rev/Fwd" class="Clust (strict)"("Visible"=w247) -> ()  [unwired: 2 in, 2 out]
            n154 = Not(x=w247) -> (.not. x?=w248:bool)
            n155 = property on="On/Off" class="Bool (strict)"("Visible"=w248, "Caption.Text"=w246) -> ()  [unwired: 2 in, 2 out]
          }
          frame "Compressor", "Digital Out" {
            w254 = FALSE ("Visible")
            # "Get direction and finish"
            n156 = property on="Test Ring" class="Ring (strict)"("Visible"=w254) -> ()  [unwired: 2 in, 2 out]
            n157 = property on="Motor" class="Clust (strict)"("Visible"=w254) -> ()  [unwired: 2 in, 2 out]
            n158 = property on="Test Slider" class="Slide (strict)"("Visible"=w254) -> ()  [unwired: 2 in, 2 out]
            n159 = property on="Rev/Fwd" class="Clust (strict)"("Visible"=FALSE) -> ()  [unwired: 2 in, 2 out]
            n160 = property on="On/Off" class="Bool (strict)"("Visible"=TRUE, "Caption.Text"=w255) -> ()  [unwired: 2 in, 2 out]
          }
          frame "Camera" {
            n161 = call <vilib>:"Get Last Path Segment.vi"("String in"=w262) -> ("String out"=w263:string)  [unwired: 10 in]
            n162 = property on="Rev/Fwd" class="Clust (strict)"("Visible"=FALSE) -> ()  [unwired: 2 in, 2 out]
            n163 = case shown="\"White Balance  **\"" w263 {
              tunnel: w262 -> [w269 w278 w287 w296 w305 _ w311]
              tunnel: w261 -> [w267 w275 w284 w293 w302 _ _]
              frame "Size  **" {
                n164 = Index Array(array=w267) -> (element=w266:cluster{string[]})  [unwired: 1 in]
                n165 = call <vilib>:"NT Read String.vi"("Name"=w269) -> ("String"=w268:string)  [unwired: 9 in, 1 out]
                n166 = property on="Test Slider" class="Slide (strict)"("Visible"=FALSE) -> ()  [unwired: 2 in, 2 out]
                n167 = property on="Test Ring" class="Ring (strict)"("Visible"=TRUE) -> ()  [unwired: 2 in, 2 out]
                n168 = Unbundle(w266) -> (w264:string[])
                n169 = Match First String(2:w264, 3:w268) -> (0:w265:i32)  [unwired: 1 out]
                n170 = property on="Test Ring" class="Ring (strict)"("Value"=w265, "Strings []"=w264) -> ()  [unwired: 2 in, 2 out]
              }
              frame "White Balance  **" {
                n171 = call <vilib>:"NT Read String.vi"("Name"=w278) -> ("String"=w277:string)  [unwired: 9 in, 1 out]
                n172 = Index Array(array=w275, index=1) -> (element=w276:cluster{string[]})
                n173 = property on="Test Slider" class="Slide (strict)"("Visible"=FALSE) -> ()  [unwired: 2 in, 2 out]
                n174 = property on="Test Ring" class="Ring (strict)"("Visible"=TRUE) -> ()  [unwired: 2 in, 2 out]
                n175 = Unbundle(w276) -> (w273:string[])
                n176 = Match First String(2:w273, 3:w277) -> (0:w272:i32)  [unwired: 1 out]
                n177 = property on="Test Ring" class="Ring (strict)"("Value"=w272, "Strings []"=w273) -> ()  [unwired: 2 in, 2 out]
              }
              frame "Exposure  **" {
                n178 = call <vilib>:"NT Read String.vi"("Name"=w287) -> ("String"=w286:string)  [unwired: 9 in, 1 out]
                n179 = Index Array(array=w284, index=2) -> (element=w285:cluster{string[]})
                n180 = property on="Test Slider" class="Slide (strict)"("Visible"=FALSE) -> ()  [unwired: 2 in, 2 out]
                n181 = property on="Test Ring" class="Ring (strict)"("Visible"=TRUE) -> ()  [unwired: 2 in, 2 out]
                n182 = Unbundle(w285) -> (w281:string[])
                n183 = Match First String(2:w281, 3:w286) -> (0:w282:i32)  [unwired: 1 out]
                n184 = property on="Test Ring" class="Ring (strict)"("Value"=w282, "Strings []"=w281) -> ()  [unwired: 2 in, 2 out]
              }
              frame "Exposure Priority  **" {
                n185 = call <vilib>:"NT Read String.vi"("Name"=w296) -> ("String"=w295:string)  [unwired: 9 in, 1 out]
                n186 = Index Array(array=w293, index=3) -> (element=w294:cluster{string[]})
                n187 = property on="Test Slider" class="Slide (strict)"("Visible"=FALSE) -> ()  [unwired: 2 in, 2 out]
                n188 = property on="Test Ring" class="Ring (strict)"("Visible"=TRUE) -> ()  [unwired: 2 in, 2 out]
                n189 = Unbundle(w294) -> (w290:string[])
                n190 = Match First String(2:w290, 3:w295) -> (0:w291:i32)  [unwired: 1 out]
                n191 = property on="Test Ring" class="Ring (strict)"("Value"=w291, "Strings []"=w290) -> ()  [unwired: 2 in, 2 out]
              }
              frame "Color Enable  **" {
                n192 = call <vilib>:"NT Read String.vi"("Name"=w305) -> ("String"=w304:string)  [unwired: 9 in, 1 out]
                n193 = Index Array(array=w302, index=4) -> (element=w303:cluster{string[]})
                n194 = property on="Test Slider" class="Slide (strict)"("Visible"=FALSE) -> ()  [unwired: 2 in, 2 out]
                n195 = property on="Test Ring" class="Ring (strict)"("Visible"=TRUE) -> ()  [unwired: 2 in, 2 out]
                n196 = Unbundle(w303) -> (w299:string[])
                n197 = Match First String(2:w299, 3:w304) -> (0:w300:i32)  [unwired: 1 out]
                n198 = property on="Test Ring" class="Ring (strict)"("Value"=w300, "Strings []"=w299) -> ()  [unwired: 2 in, 2 out]
              }
              frame Default {
                n199 = property on="Test Slider" class="Slide (strict)"("Visible"=FALSE) -> ()  [unwired: 2 in, 2 out]
                n200 = property on="Test Ring" class="Ring (strict)"("Visible"=FALSE) -> ()  [unwired: 2 in, 2 out]
              }
              frame "Brightness  **", "Color Level  **", "Compression  **", "FPS  **", "Sharpness  **" {
                n201 = call <vilib>:"NT Read Number.vi"("Name"=w311) -> ("Numeric"=w310:dbl)  [unwired: 9 in, 1 out]
                n202 = property on="Test Ring" class="Ring (strict)"("Visible"=FALSE) -> ()  [unwired: 2 in, 2 out]
                n203 = property on="Test Slider" class="Slide (strict)"("Visible"=TRUE, "Scale.Maximum"=100.0 ("Scale.Range:Maximum")) -> ()  [unwired: 2 in, 2 out]
                n204 = local write "Test Slider"(w310) -> ()
              }
            }
            n205 = property on="On/Off" class="Bool (strict)"("Visible"=FALSE) -> ()  [unwired: 2 in, 2 out]
            n206 = property on="Motor" class="Clust (strict)"("Visible"=FALSE) -> ()  [unwired: 2 in, 2 out]
          }
        }
      }
      event "Test Name": Mouse Enter {
        # "Populate the ring with the list of tests"
        n207 = event-data() -> ()  [unwired: 1 in, 1 out]
        n208 = call <vilib>:"NT Read String Array.vi"("Name"="TestMode/TestList") -> ("String Array"=w319:string[])  [unwired: 9 in, 1 out]
        n209 = Build Array (concatenate)("Select the test to run...", w319) -> (w318:string[])
        n210 = property on="Test Name" class="Ring (strict)"("Strings []"=w318) -> ()  [unwired: 2 in, 2 out]
      }
      event "Test Name": Value Change {
        w321 = FALSE ("Visible")
        # "Tell the robot the test name to run"
        n211 = event-data() -> ("NewVal"=w325:u16)  [unwired: 1 in]
        n212 = property on="Test Ring" class="Ring (strict)"("Visible"=w321) -> ()  [unwired: 2 in, 2 out]
        n213 = property on="Motor" class="Clust (strict)"("Visible"=w321) -> ()  [unwired: 2 in, 2 out]
        n214 = property on="Test Slider" class="Slide (strict)"("Visible"=w321) -> ()  [unwired: 2 in, 2 out]
        n215 = property on="On/Off" class="Bool (strict)"("Visible"=w321) -> ()  [unwired: 2 in, 2 out]
        n216 = property on="Rev/Fwd" class="Clust (strict)"("Visible"=w321) -> ()  [unwired: 2 in, 2 out]
        n217 = local write "Progress"(T8 {"Test Progress"=0, "Test Progress Text"=""} ("Progress")) -> ()
        n218 = property on="Progress" class="Clust (strict)"("Visible"=TRUE) -> ()  [unwired: 2 in, 2 out]
        n219 = property on="Test Name" class="Ring (strict)"() -> ("Strings []"=w326:string[])  [unwired: 2 in, 2 out]
        n220 = Index Array(array=w326, index=w325) -> (element=w324:string)
        n221 = call <vilib>:"NT Write String.vi"("String"=w324, "Name"="TestMode/TestName") -> ()  [unwired: 9 in, 1 out]
      }
      event "Listbox": Double Click {
        # "Shift clears all"
        # "Update symbols on the listbox"
        n222 = event-data() -> ("PlatMods.Shift"=w329:bool, "Row"=w331:i32)  [unwired: 1 in]
        n223 = case shown="True" w329 {
          tunnel: w331 -> [w335 _]
          tunnel: 1 -> [w334 _]
          frame False {
            n224 = property on="Listbox" class="LstBox (strict)"() -> ("Item Symbols"=w333:i32[])  [unwired: 2 in, 2 out]
            n225 = Replace Array Subset(array=w333, new element=w334, index=w335) -> (w332:i32[])
            n226 = property on="Listbox" class="LstBox (strict)"("Item Symbols"=w332) -> ()  [unwired: 2 in, 2 out]
          }
          frame True {
            w336 = 0 ("Top Row")
            n227 = property on="Listbox" class="LstBox (strict)"() -> ("Number of Rows"=w338:u32)  [unwired: 2 in, 2 out]
            n228 = Initialize Array(0, w338) -> (w337:i32[])
            n229 = property on="Listbox" class="LstBox (strict)"("Top Row"=w336, "Value"=w336, "Item Symbols"=w337) -> ()  [unwired: 2 in, 2 out]
          }
        }
      }
      event "Listbox": Key Down {
        # "Update symbols on the listbox\nLeft and right keys check and uncheck"
        n230 = event-data() -> ("VKey"=w342:T22)  [unwired: 1 in]
        n231 = case shown="\"Left\", \"Right\"" w342 {
          selector: w342 -> [w347 _]
          tunnel: eventvkey."Left" ("VKey") -> [w345 _]
          frame "Left", "Right" {
            n232 = Equal?(x=w345, y=w347) -> (x = y?=w346:bool)
            n233 = Select(t=0, s=w346, f=1) -> (s? t:f=w348:i32)
            n234 = property on="Listbox" class="LstBox (strict)"() -> ("Item Symbols"=w351:i32[])  [unwired: 2 in, 2 out]
            n235 = Replace Array Subset(array=w351, new element=w348, index="Listbox") -> (w350:i32[])
            n236 = property on="Listbox" class="LstBox (strict)"("Item Symbols"=w350) -> ()  [unwired: 2 in, 2 out]
          }
          frame Default {
          }
        }
      }
      event "DB Camera Config": Value Change {
        # "Show or hide the cluster of controls, store in ini file"
        n237 = event-data() -> ("NewVal"=w355:bool)  [unwired: 1 in]
        n238 = case shown="False" w355 {
          tunnel: w354 -> [w364 _]
          tunnel: [w357 w375] -> w353
          tunnel: w352 -> [w356 w375]
          frame False {
            w371 = "Camera"
            w374 = FALSE ("Visible")
            n239 = property on="Camera Settings" class="Clust (strict)"("Visible"=w374) -> ()  [unwired: 2 in, 2 out]
            n240 = local write "DB Camera Config"(w374) -> ()
            n241 = local read "Camera Settings"() -> (w363:T2)
            n242 = Index Array(array=w364) -> (element=w367:cluster{string[]})  [unwired: 1 in]
            n243 = Unbundle(w367) -> (w366:string[])
            n244 = Unbundle(w363) -> ("Frame Rate"=w362:i32, "Compression"=w361:i32, "Size"=w365:u16)
            n245 = Index Array(array=w366, index=w365) -> (element=w360:string)
            n246 = call-poly <vilib>:"Write Key.vi"("section"=w371, "value"=w360, "key"="Size", "refnum"=w356) -> ("refnum out"=w373:T13)  [unwired: 2 in, 5 out]
            n247 = call-poly <vilib>:"Write Key.vi"("section"=w371, "value"=w362, "key"="FrameRate", "refnum"=w373) -> ("refnum out"=w372:T13)  [unwired: 1 in, 6 out]
            n248 = call-poly <vilib>:"Write Key.vi"("section"=w371, "value"=w361, "key"="Compression", "refnum"=w372) -> ("refnum out"=w358:T13)  [unwired: 1 in, 6 out]
            n249 = call <vilib>:"Close Config Data.vi"("refnum"=w358) -> ("file path"=w359:path)  [unwired: 2 in, 8 out]
            n250 = call <vilib>:"Open Config Data.vi"("configuration file path"=w359) -> ("refnum"=w357:T13)  [unwired: 8 in, 2 out]
          }
          frame True {
            n251 = property on="Camera Settings" class="Clust (strict)"("Visible"=TRUE) -> ()  [unwired: 2 in, 2 out]
          }
        }
      }
      event "Camera Settings": Value Change {
        # "Update summary string when any elements of DB camera change"
        n252 = event-data() -> ("NewVal"=w388:T2)  [unwired: 1 in]
        n253 = Index Array(array=w384) -> (element=w383:cluster{string[]})  [unwired: 1 in]
        n254 = Unbundle(w383) -> (w382:string[])
        n255 = Unbundle(w388) -> ("Frame Rate"=w379:i32, "Compression"=w378:i32, "Size"=w381:u16)
        n256 = Index Array(array=w382, index=w381) -> (element=w380:string)
        n257 = Format Into String(format string="%s   %dfps   %d%%", w380, w379, w378) -> (resulting string=w385:string)  [unwired: 2 in, 1 out]
        n258 = Build Array(w385) -> (w386:string[])
        n259 = property on="DB Camera Config" class="Bool (strict)"("Strings [4]"=w386) -> ()  [unwired: 2 in, 2 out]
      }
      event "Motor.Enable": Value Change {
        # "When the test mode otor enable helper is set, update that\ntree row item's value"
        n260 = event-data() -> ("NewVal"=w394:bool)  [unwired: 1 in]
        n261 = Unbundle("Motor") -> ("Value"=w393:dbl)  [unwired: 1 out]
        n262 = Select(t=w393, s=w394, f=0.0) -> (s? t:f=w391:dbl)
        n263 = call <vilib>:"NT Write Number.vi"("Numeric"=w391, "Name"=w390) -> ()  [unwired: 9 in, 1 out]
      }
      event "Test Slider": Value Change {
        # "When the test mode slider helper is set, update that\ntree row item's value"
        n264 = event-data() -> ("NewVal"=w397:dbl)  [unwired: 1 in]
        n265 = call <vilib>:"NT Write Number.vi"("Numeric"=w397, "Name"=w398) -> ()  [unwired: 9 in, 1 out]
      }
      event "On/Off": Value Change {
        # "When the test mode on/off helper value is set, update that\ntree row item's value"
        n266 = event-data() -> ("NewVal"=w402:bool)  [unwired: 1 in]
        n267 = Boolean To (0,1)(Boolean=w402) -> (0, 1=w401:i16)
        n268 = call <vilib>:"NT Write Number.vi"("Numeric"=w401, "Name"=w400) -> ()  [unwired: 9 in, 1 out]
      }
      event "Rev/Fwd": Value Change {
        # "When the test mode helper value for relays is set, update that\ntree row item's value"
        n269 = event-data() -> ("NewVal.Forward"=w410:bool, "NewVal.Reverse"=w409:bool)  [unwired: 1 in]
        n270 = Boolean To (0,1)(Boolean=w409) -> (0, 1=w408:i16)
        n271 = Boolean To (0,1)(Boolean=w410) -> (0, 1=w406:i16)
        n272 = Negate(x=w408) -> (-x=w407:i16)
        n273 = Add(x=w406, y=w407) -> (x+y=w405:i16)
        n274 = call <vilib>:"NT Write Number.vi"("Numeric"=w405, "Name"=w404) -> ()  [unwired: 9 in, 1 out]
      }
      event "Test Ring": Value Change {
        # "When a test mode helper value is selected from the ring,\nset the tree item's variable to the string value"
        n275 = event-data() -> ("NewVal"=w414:u16)  [unwired: 1 in]
        n276 = property on="Test Ring" class="Ring (strict)"() -> ("Strings []"=w415:string[])  [unwired: 2 in, 2 out]
        n277 = Index Array(array=w415, index=w414) -> (element=w413:string)
        n278 = call <vilib>:"NT Write String.vi"("String"=w413, "Name"=w412) -> ()  [unwired: 9 in, 1 out]
      }
      event "Rec Mode": Value Change {
        # "Update globals for recording mode and path to read log from.\nClear when logging and let NetworkTables set path for vision to\nuse."
        n279 = event-data() -> ("NewVal"=w425:enum32{"Stop", "Record", "Playback"})  [unwired: 1 in]
        n280 = global write "WPI_DashboardLogging Global.vi" "Logging Filename"(path "") -> ()
        n281 = global write "WPI_DashboardLogging Global.vi" "Recording"(w425) -> ()
        n282 = case shown="\"Playback\"" w425 {
          tunnel: w424 -> [_ w427 w435]
          tunnel: [_ _ w434] -> w421
          tunnel: [_ _ w433] -> _
          tunnel: w419 -> [_ _ w431]
          tunnel: cluster{i32, i32} {-250, 170} -> [_ _ w430]
          tunnel: [_ _ T23 {"Image Size"=TRUE, "Image Type"=TRUE, "Pixel Value"=TRUE, "ROI Information"=TRUE, "Zoom Factor"=FALSE} ("Image Information Shown:All Elements")] -> w417
          tunnel: [_ _ TRUE ("Zoom Factor")] -> w416
          frame Default {
          }
          frame "Stop", "Record" {
            # "Place Window too"
            n283 = invoke class="VI" method="FP.Close"(reference=w427) -> (reference out=w426:refnum<vi>)  [unwired: 2 in, 2 out]
            n284 = invoke class="VI" method="Abort VI"(reference=w426) -> ()  [unwired: 2 in, 3 out]
          }
          frame "Playback" {
            n285 = call "Open Playback Panel.vi"("Offset"=w430, "DB VI Ref"=w431, "Playback in"=w435) -> ("Playback out"=w432:refnum<vi>)  [unwired: 8 in]
            n286 = register-events(w432) -> (reference out=w434:refnum<event-registration>, error out=w433:errorcluster)  [unwired: 2 in]
          }
        }
        n287 = property on="Camera Image" class="ImageControl"("Image Information Shown"=w417, "Image Information Visible"=w416) -> ()  [unwired: 2 in, 2 out]
        n288 = call <vilib>:"WPI_DashboardNT Log FieldName Cache.vi"("Operation"=enum16{"Lookup/Add", "Index", "Clear"}."Clear") -> ()  [unwired: 8 in, 3 out]
      }
      event Panel Close {
        w436 = enum32{"Stop", "Record", "Playback"}."Stop" ("Rec Mode")
        # "Playback window has been closed, abort"
        n289 = event-data() -> ()  [unwired: 1 in, 4 out]
        n290 = local write "Rec Mode"(w436) -> ()
        n291 = global write "WPI_DashboardLogging Global.vi" "Recording"(w436) -> ()
      }
      event Panel Close {
        # "Abort playback window and ourself"
        n292 = event-data() -> ()  [unwired: 1 in, 4 out]
        n293 = invoke class="VI" method="FP.Close"(reference=w441) -> (reference out=w440:refnum<vi>)  [unwired: 2 in, 2 out]
        n294 = invoke class="VI" method="Abort VI"(reference=w440) -> (error out=w439:errorcluster)  [unwired: 2 in, 2 out]
        n295 = invoke class="VI" method="Abort VI"(error in=w439) -> ()  [unwired: 2 in, 3 out]
      }
      event "Vision": Value Change {
        # "Enable/Disable Compression slider.\nHW USB is hard-coded into the camera"
        n296 = event-data() -> ("NewVal"=w447:u16)  [unwired: 1 in]
        n297 = Equal?(x=w447, y=u32 2 ("milliseconds to wait")) -> (x = y?=w445:bool)
        n298 = Select(t=T24."Disabled and Grayed Out" ("Disabled"), s=w445, f=T24."Enabled" ("Disabled")) -> (s? t:f=w442:T24)
        n299 = property on="Compression" class="Slide (strict)"("DisabledEnum"=w442) -> ()  [unwired: 2 in, 2 out]
      }
    }
  }
